vi "DAQ Close.vi"(8 "error in":errorcluster, 11 "DAQmx Task In":refnum<k21>) -> (0 "error out":errorcluster)   [LabVIEW 2020]
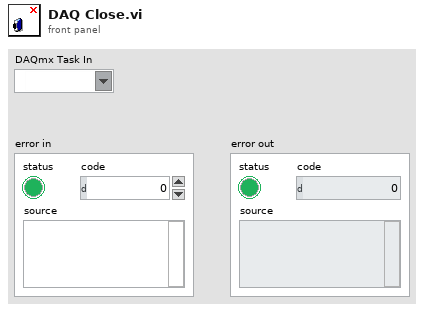
[diagram p1: front panel]
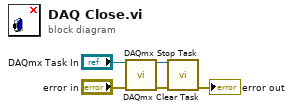
[diagram p0: block diagram]
diagram:
  n1 = call <vilib>:"DAQmx Stop Task.vi"("task/channels in"="DAQmx Task In", "error in"="error in") -> ("task out"=w2:refnum<k21>, "error out"=w5:errorcluster)  [unwired: 12 in]
  n2 = call <vilib>:"DAQmx Clear Task.vi"("task in"=w2, "error in"=w5) -> ("error out"=→"error out":errorcluster)  [unwired: 13 in]
